vi "test vi.vi"() -> ()   [LabVIEW 2013]
uses:
  <vilib>/Instr/_visa.llb/VISA Open Access Mode.ctl
panel:
  out "unsigned byte array":u8[](array[numeric])
  out "Array":string[](array[string])
  in  "VISA resource name":refnum<visa-resource-name>
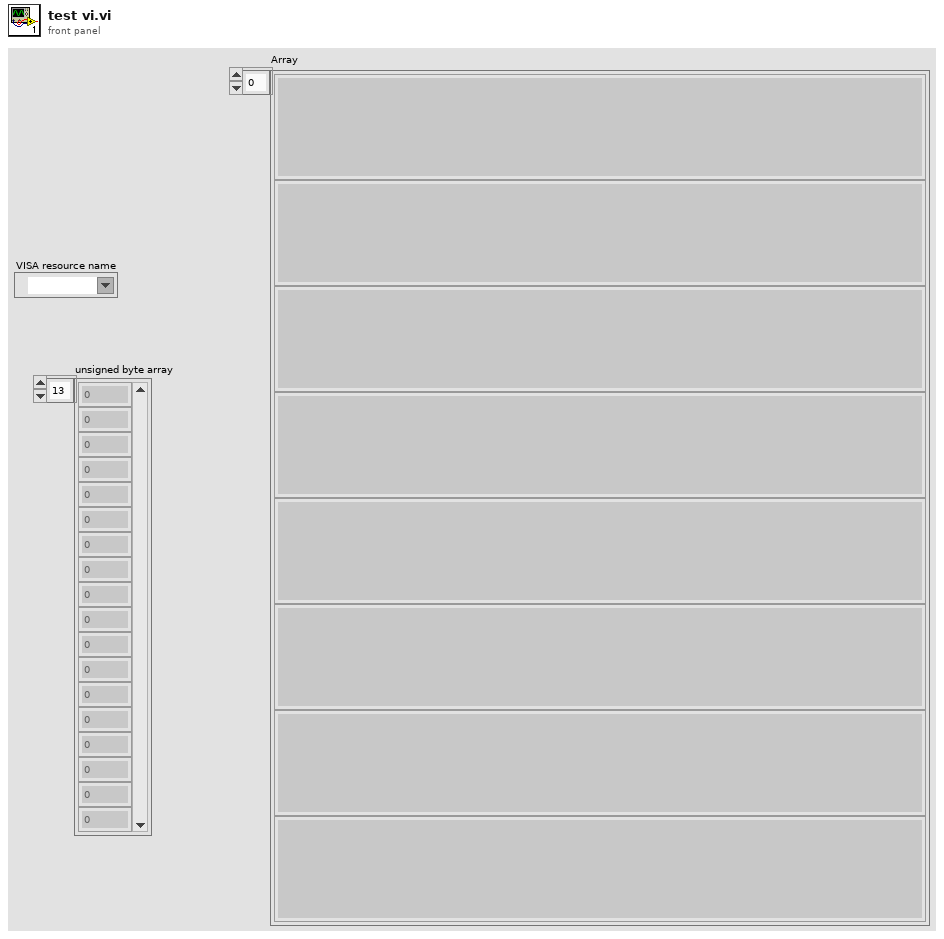
[diagram p1: front panel]
types:
  T1 = typedef "VISA Open Access Mode.ctl" = u32
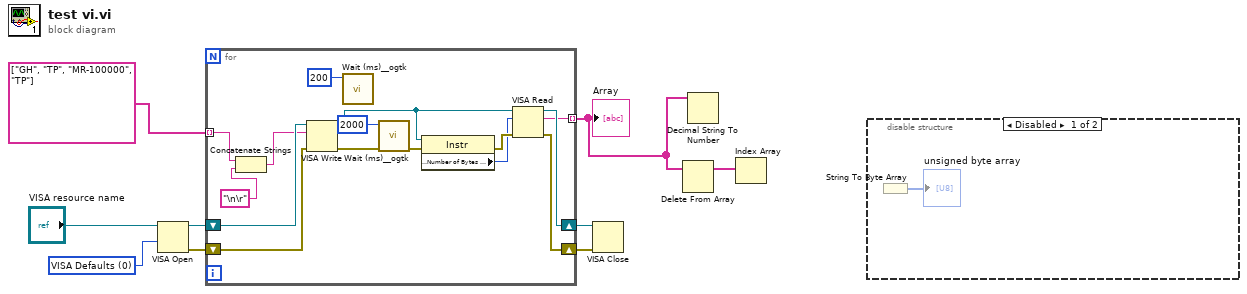
[diagram p0: block diagram]
diagram:
  w6 = T1 0 items=["VISA Defaults"=0, "Exclusive Lock"=1, "Load Configured Settings"=4] ("Access Mode")
  n1 = VISA Open(access mode=w6, VISA resource name="VISA resource name") -> (VISA resource name=w8:refnum<visa-resource-name>, error out=w7:errorcluster)  [unwired: 3 in]
  n2 = for {
    tunnel: string[] ["GH", "TP", "MR-100000", "TP"] -> [w12] mode=indexing
    shift-right: [w20] -> w4
    shift-left: w7 -> [w23]
    shift-right: [w21] -> w3
    shift-left: w8 -> [w24]
    tunnel: [w14] -> w2 mode=indexing
    n3 = Concatenate Strings(w12, "\n\r") -> (w10:string)
    n4 = VISA Write(VISA resource name=w24, write buffer=w10, error in (no error)=w23) -> (VISA resource name out=w17:refnum<visa-resource-name>, error out=w19:errorcluster)  [unwired: 1 out]
    n5 = call <userlib>:"Wait (ms)__ogtk.vi"("milliseconds to wait"=u32 200) -> ()  [unwired: 9 in, 2 out]
    n6 = call <userlib>:"Wait (ms)__ogtk.vi"("error in (no error)"=w19, "milliseconds to wait"=u32 2000) -> ("error out"=w16:errorcluster)  [unwired: 8 in, 1 out]
    n7 = property class="Instr"(reference=w17, error in=w16) -> (error out=w18:errorcluster, "Serial Settings:Number of Bytes at Serial Port"=w13:u32)  [unwired: 1 out]
    n8 = VISA Read(VISA resource name=w17, byte count=w13, error in (no error)=w18) -> (VISA resource name out=w21:refnum<visa-resource-name>, read buffer=w14:string, error out=w20:errorcluster)  [unwired: 1 out]
  }
  "Array" <- w2
  n9 = VISA Close(VISA resource name=w3, error in (no error)=w4) -> ()  [unwired: 1 out]
  n10 = Delete From Array(array=w2) -> (array with subset deleted=w1:string[])  [unwired: 2 in, 1 out]
  n11 = Decimal String To Number(string=w2) -> ()  [unwired: 2 in, 2 out]
  n12 = Index Array(array=w1) -> ()  [unwired: 1 in, 1 out]
  n13 = disable-structure shown="Disabled" {
    frame Disabled {
      n14 = String To Byte Array() -> (unsigned byte array=→"unsigned byte array":u8[])  [unwired: 1 in]
    }
    frame Enabled {
    }
  }
